vi "LocalAddress.vi"() -> (1 "IP Address (xx.xx.xx.xx)":string, 2 "IP Address (name.domain.com)":string, 3 "net address":u32 format="%x")   [LabVIEW 2010]
doc: "The String to IP function will return the local machines IP address as number if the input is left empty. The bytes of the number correspond to the parts of the IP address. This can be converted to a string by using the IP to String function."
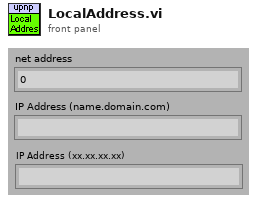
[diagram p1: front panel]
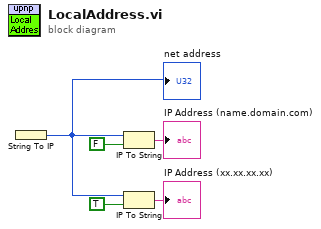
[diagram p0: block diagram]
diagram:
  n1 = String To IP() -> (0:w1:u32)  [unwired: 1 out]
  "net address" <- w1
  n2 = IP To String(1:FALSE ("dot notation? (F)"), 2:w1) -> (0:→"IP Address (name.domain.com)":string)
  n3 = IP To String(1:TRUE ("dot notation? (F)"), 2:w1) -> (0:→"IP Address (xx.xx.xx.xx)":string)
